vi "GDSLvIcon_CalcWordsPerRowSubVI.vi"(2 "Pixel width":i32, 3 "wordData":T1[](array[typedef]), 4 "EnterCharAtTheseLocations":i32[](array[numeric]), 5 "error in (no error)":errorcluster, 6 "StartWordIndex":i32) -> (15 "Words":i32, 16 "RowNeedsToBeCompressed":bool, 19 "error out":errorcluster)   [LabVIEW 2016]
uses:
  <resource>/Framework/Providers/Open_GDS/ClassProviders/Common/LvIcon_class/subvis/GDSLvIcon_WordDataType.ctl
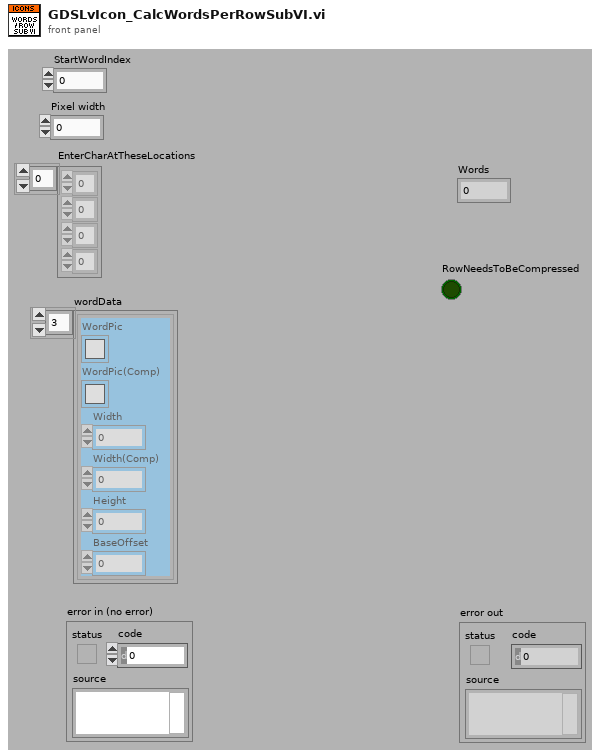
[diagram p1: front panel]
types:
  T1 = typedef "GDSLvIcon_WordDataType.ctl" = cluster{"WordPic":bool[][], "WordPic(Comp)":bool[][], "Width":i32, "Width(Comp)":i32, "Height":i32, "BaseOffset":i32}
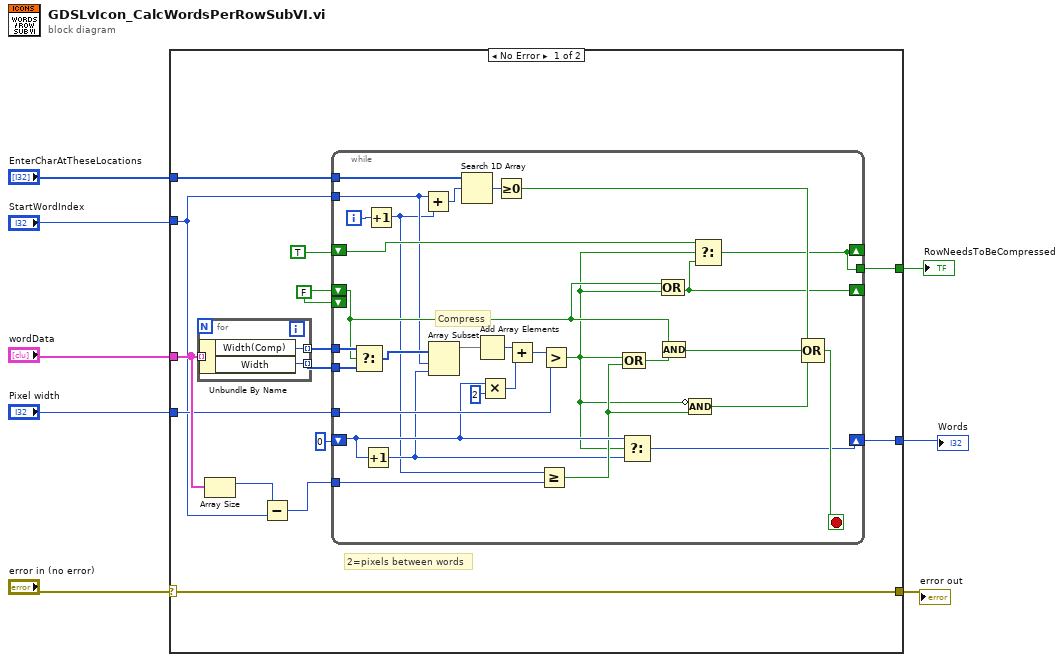
[diagram p0: block diagram]
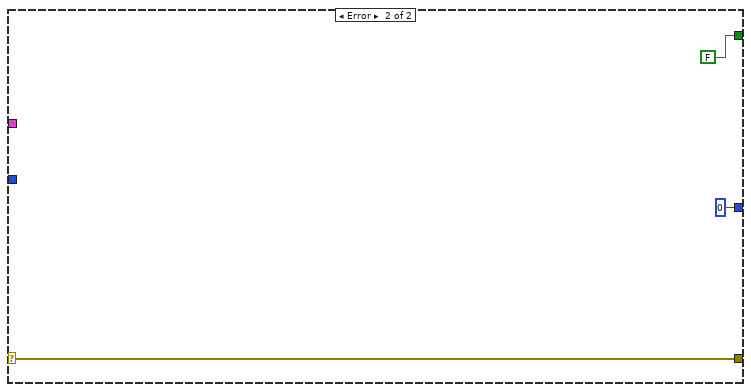
[diagram p2: hidden frame]
diagram:
  n1 = case shown="No Error" "error in (no error)" {
    selector: "error in (no error)" -> [w22 w58]
    tunnel: [w22 w58] -> w7
    tunnel: "wordData" -> [w21 _]
    tunnel: "StartWordIndex" -> [w11 _]
    tunnel: "Pixel width" -> [w18 _]
    tunnel: "EnterCharAtTheseLocations" -> [w17 _]
    tunnel: [w15 0 ("y")] -> w3
    tunnel: [w14 FALSE] -> w2
    frame No Error {
      w13 = FALSE
      # "2=pixels between words"
      n2 = for {
        tunnel: [w55] -> w20 mode=indexing
        tunnel: [w54] -> w19 mode=indexing
        tunnel: w21 -> [w53] mode=indexing
        n3 = Unbundle By Name(w53) -> ("Width(Comp)"=w55:i32, "Width"=w54:i32)
      }
      n4 = Array Size(array=w21) -> (size(s)=w10:i32)
      n5 = Subtract(x=w10, y=w11) -> (x-y=w9:i32)
      n6 = while {
        shift-left: TRUE -> [w32]
        shift-right: [w31] -> _
        tunnel: w11 -> [w25]
        tunnel: [w31] -> w14
        tunnel: w9 -> [w40]
        shift-left: w13 -> [_]
        shift-left: 0 ("y") -> [w34]
        shift-right: [w37] -> w15
        tunnel: w17 -> [w47]
        tunnel: w18 -> [w48]
        tunnel: w19 -> [w50]
        tunnel: w20 -> [w51]
        shift-left: w13 -> [w30]
        shift-right: [w29] -> _
        i -> [w43]
        stop <- w44 stop-if-true
        # "Compress"
        n7 = Select(t=w51, s=w30, f=w50) -> (s? t:f=w39:i32[])
        n8 = Increment(x=w34) -> (x+1=w24:i32)
        n9 = Increment(x=w43) -> (x+1=w23:i32)
        n10 = Add(x=w25, y=w23) -> (x+y=w33:i32)
        n11 = Array Subset(array=w39, index=w25, length=w24) -> (w38:i32[])
        n12 = Search 1D Array(1D array=w47, element=w33) -> (index of element=w46:i32)  [unwired: 1 in]
        n13 = Add Array Elements(numeric array=w38) -> (sum=w35:i32)
        n14 = Multiply(x=w34, y=2) -> (x*y=w36:i32)
        n15 = Greater Or Equal To 0?(x=w46) -> (x >= 0?=w45:bool)
        n16 = Add(x=w35, y=w36) -> (x+y=w49:i32)
        n17 = Greater Or Equal?(x=w23, y=w40) -> (x >= y?=w28:bool)
        n18 = Greater?(x=w49, y=w48) -> (0:w27:bool)
        n19 = Select(t=w34, s=w27, f=w24) -> (s? t:f=w37:i32)
        n20 = Compound Arithmetic op=OR(w27, w28) -> (w42:bool)
        n21 = Compound Arithmetic op=OR(w30, w27) -> (w29:bool)
        n22 = Compound Arithmetic op=AND(w30, w42) -> (w41:bool)
        n23 = Compound Arithmetic op=AND(invert w27, w28) -> (w26:bool)
        n24 = Select(t=w32, s=w27, f=w29) -> (s? t:f=w31:bool)
        n25 = Compound Arithmetic op=OR(w45, w41, w26) -> (w44:bool)
      }
    }
    frame Error {
    }
  }
  "error out" <- w7
  "Words" <- w3
  "RowNeedsToBeCompressed" <- w2
